vi "Send Commands to MC.vi"(7 "Pause Motors":bool, 8 "error in":errorcluster, 9 "Prev MC cmd":cluster{"cmd a":i16, "cmd b":i16}, 10 "Motor Command":T1, 11 "MC refrence in":refnum<visa-resource-name>) -> (0 "error out":errorcluster, 1 "New MC cmd":cluster{"cmd a":i16, "cmd b":i16}, 3 "MC refrence out":refnum<visa-resource-name>, 5 "MC Commands":cluster{"Cmd A":string, "Cmd B":string})   [LabVIEW 2009]
uses:
  Remote Control/Motor Command.ctl
panel:
  in  "speed step":i16=5
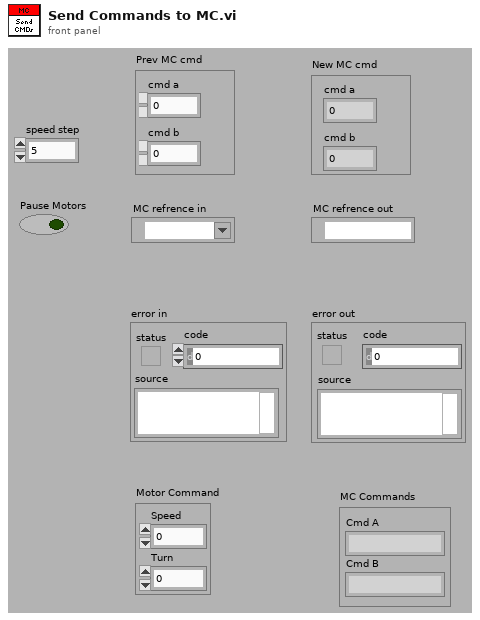
[diagram p1: front panel]
types:
  T1 = typedef "Motor Command.ctl" = cluster{"Speed":i16, "Turn":i16}
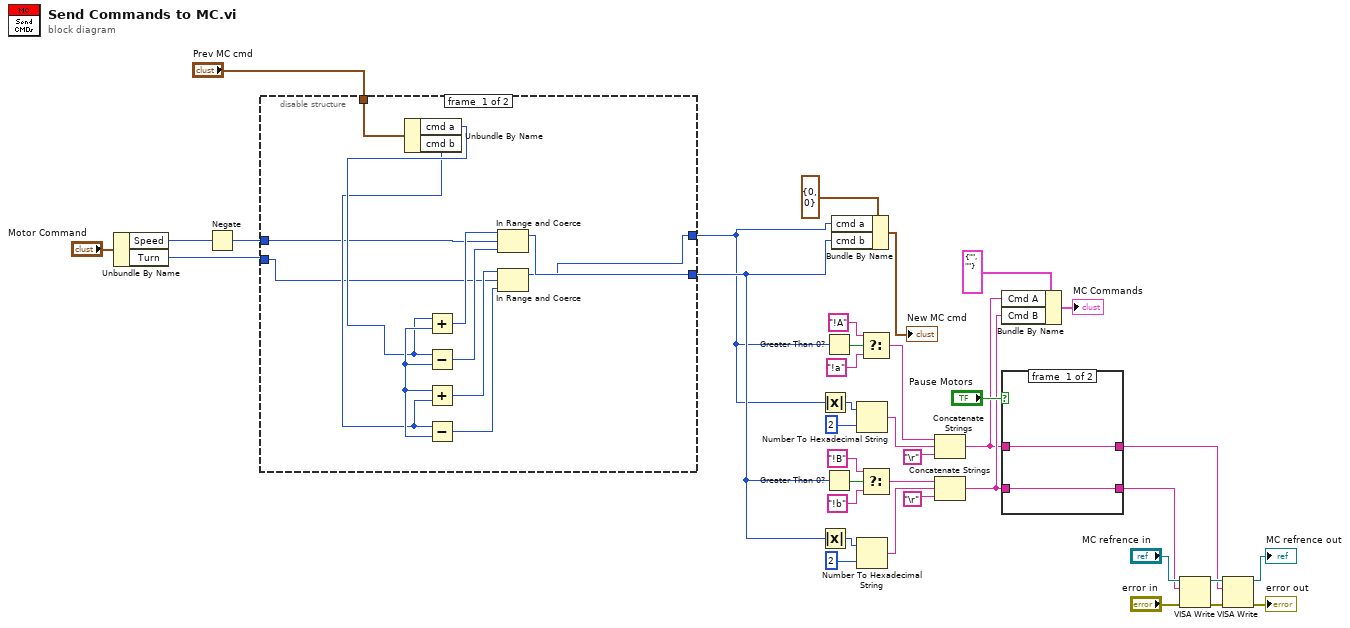
[diagram p0: block diagram]
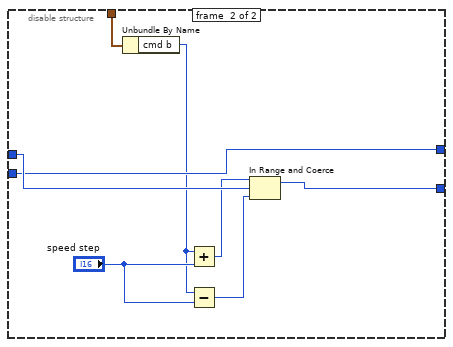
[diagram p2: hidden frame]
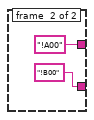
[diagram p3: hidden frame]
diagram:
  n1 = Unbundle By Name("Motor Command") -> ("Speed"=w12:i16, "Turn"=w1:i16)
  n2 = Negate(x=w12) -> (-x=w2:i16)
  n3 = disable-structure shown="Enabled" {
    disable-tunnel: w2 -> [w42 w58]
    disable-tunnel: w1 -> [w41 w57]
    disable-tunnel: [w40 w56] -> w7
    disable-tunnel: [w39 w57] -> w6
    disable-tunnel: "Prev MC cmd" -> [w43 w55]
    frame #0 {
      n4 = Unbundle By Name(w43) -> ("cmd a"=w45:i16, "cmd b"=w44:i16)
      n5 = Add(x=w45) -> (y=w46:i16, x+y=w50:i16)
      n6 = Subtract(x=w45, y=w46) -> (x-y=w48:i16)
      n7 = Add(x=w46, y=w44) -> (x+y=w49:i16)
      n8 = Subtract(x=w44, y=w46) -> (x-y=w47:i16)
      n9 = In Range and Coerce(upper limit=w50, x=w42, lower limit=w48) -> (coerced(x)=w40:i16)  [unwired: 1 out]
      n10 = In Range and Coerce(upper limit=w49, x=w41, lower limit=w47) -> (coerced(x)=w39:i16)  [unwired: 1 out]
    }
    frame #1 {
      n11 = Unbundle By Name(w55) -> ("cmd b"=w53:i16)
      n12 = Add(x=w53, y="speed step") -> (x+y=w52:i16)
      n13 = Subtract(x=w53, y="speed step") -> (x-y=w51:i16)
      n14 = In Range and Coerce(upper limit=w52, x=w58, lower limit=w51) -> (coerced(x)=w56:i16)  [unwired: 1 out]
    }
  }
  n15 = Absolute Value(x=w6) -> (abs(x)=w30:i16)
  n16 = Absolute Value(x=w7) -> (abs(x)=w31:i16)
  n17 = Greater Than 0?(x=w6) -> (x > 0?=w22:bool)
  n18 = Greater Than 0?(x=w7) -> (x > 0?=w27:bool)
  n19 = Bundle By Name(cluster=cluster{"cmd a":i16, "cmd b":i16} {"cmd a"=0, "cmd b"=0} ("Prev MC cmd"), "cmd a"=w6, "cmd b"=w7) -> (→"New MC cmd":cluster{"cmd a":i16, "cmd b":i16})
  n20 = Number To Hexadecimal String(1:i16 2 ("width (-)"), 2:w30) -> (0:w18:string)
  n21 = Number To Hexadecimal String(1:i16 2 ("width (-)"), 2:w31) -> (0:w20:string)
  n22 = Select(t="!A", s=w22, f="!a") -> (s? t:f=w19:string)
  n23 = Select(t="!B", s=w27, f="!b") -> (s? t:f=w21:string)
  n24 = Concatenate Strings(w19, w18, "\r") -> (w10:string)
  n25 = Concatenate Strings(w21, w20, "\r") -> (w11:string)
  n26 = Bundle By Name(cluster=cluster{"Cmd A":string, "Cmd B":string} {"Cmd A"="", "Cmd B"=""} ("MC Commands"), "Cmd A"=w10, "Cmd B"=w11) -> (→"MC Commands":cluster{"Cmd A":string, "Cmd B":string})
  n27 = case shown="True" "Pause Motors" {
    tunnel: w10 -> [w59 _]
    tunnel: w11 -> [w60 _]
    tunnel: [w60 "!B00" ("Left motor command")] -> w14
    tunnel: [w59 "!A00" ("Left motor command")] -> w15
    frame #0 {
    }
    frame #1 {
    }
  }
  n28 = VISA Write(VISA resource name="MC refrence in", write buffer=w14, error in (no error)="error in") -> (VISA resource name out=w38:refnum<visa-resource-name>, error out=w37:errorcluster)  [unwired: 1 out]
  n29 = VISA Write(VISA resource name=w38, write buffer=w15, error in (no error)=w37) -> (VISA resource name out=→"MC refrence out":refnum<visa-resource-name>, error out=→"error out":errorcluster)  [unwired: 1 out]
